vi "Insert Start Message.vi"(8 "error in (no error)":errorcluster, 10 "Start Time":timestamp, 11 "BehaviorData in":refnum<class "BehaviorData.lvclass">) -> (0 "error out":errorcluster, 3 "BehaviorData out":refnum<class "BehaviorData.lvclass">)   [LabVIEW 2010, in "BehaviorData.lvclass"]
uses:
  BehaviorData.lvclass
  Database/BehPrimary.ctl
  AcquireTraces/AcquireTraces.lvclass
  Database/StimulationPrimary.ctl
  <vilib>/addons/database/NI_Database_API.lvlib
  AcquistionObject/AcquistionObject.lvclass
panel:
  out "BehPK":T1
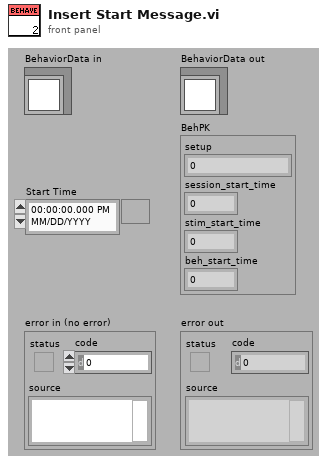
[diagram p1: front panel]
types:
  T1 = typedef "BehPrimary.ctl" = cluster{"setup":u8, "session_start_time":dbl, "stim_start_time":dbl, "beh_start_time":dbl}
  T2 = cluster{"setup":u8, "session_start_time":dbl, "stim_start_time":dbl, "beh_start_time":dbl, "beh_path":path, "beh_traces_type":string}
  T3 = typedef "NI_Database_API.lvlib/Conn ObjectReference.ctl" = refnum<k1>
  T4 = typedef "StimulationPrimary.ctl" = cluster{"setup":u8, "session_start_time":dbl, "stim_start_time":dbl}
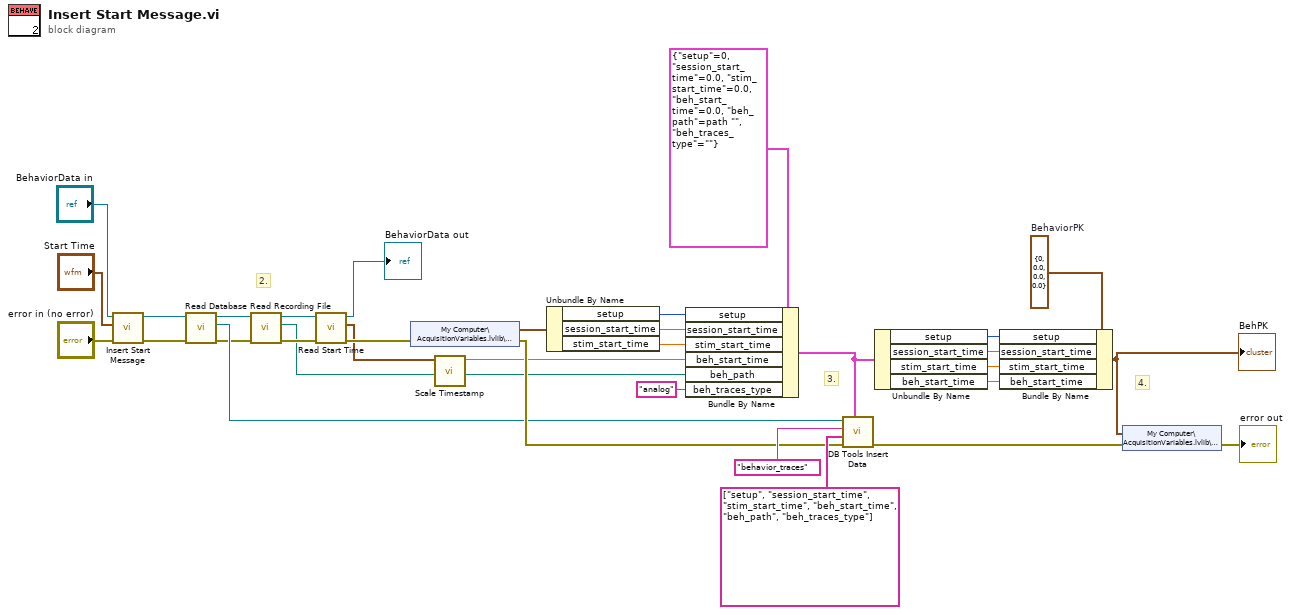
[diagram p0: block diagram]
diagram:
  w14 = T1 {"setup"=0, "session_start_time"=0.0, "stim_start_time"=0.0, "beh_start_time"=0.0}  # BehaviorPK
  # "4."
  # "2."
  # "3."
  n1 = call-parent "Insert Start Message.vi"("error in (no error)"="error in (no error)", "Start Time"="Start Time", "AcquireTraces in"="BehaviorData in") -> ("error out"=w10:errorcluster, "AcquireTraces out"=w11:refnum<class "BehaviorData.lvclass">)  [unwired: 7 in]
  n2 = call-dynamic "Read Database.vi"("error in (no error)"=w10, "AcquistionObject in"=w11) -> ("error out"=w13:errorcluster, "reference"=w17:T3, "AcquistionObject out"=w12:refnum<class "BehaviorData.lvclass">)  [unwired: 7 in]
  n3 = call-dynamic "Read Recording File.vi"("error in (no error)"=w13, "AcquistionObject in"=w12) -> ("error out"=w18:errorcluster, "Recording File"=w6:path, "AcquistionObject out"=w19:refnum<class "BehaviorData.lvclass">)  [unwired: 7 in]
  n4 = call-dynamic "Read Start Time.vi"("error in (no error)"=w18, "AcquistionObject in"=w19) -> ("error out"=w9:errorcluster, "Start Time"=w3:timestamp, "AcquistionObject out"=→"BehaviorData out":refnum<class "BehaviorData.lvclass">)  [unwired: 7 in]
  n5 = shared-variable "My Computer\\AcquisitionVariables.lvlib\\StimulationPK"(error in=w9) -> (w4:T4, error out=w22:errorcluster)
  n6 = call "Scale Timestamp.vi"("Time Stamp"=w3) -> ("Scaled timestamp"=w2:dbl)  [unwired: 10 in]
  n7 = Unbundle By Name(w4) -> ("setup"=w28:u8, "session_start_time"=w27:dbl, "stim_start_time"=w7:dbl)
  n8 = Bundle By Name(cluster=T2 {"setup"=0, "session_start_time"=0.0, "stim_start_time"=0.0, "beh_start_time"=0.0, "beh_path"=path "", "beh_traces_type"=""} ("Cluster"), "setup"=w28, "session_start_time"=w27, "stim_start_time"=w7, "beh_start_time"=w2, "beh_path"=w6, "beh_traces_type"="analog") -> (w26:T2)
  n9 = call <vilib>:"DB Tools Insert Data.vi"("data"=w26, "error in (no error)"=w22, "columns"=string[] ["setup", "session_start_time", "stim_start_time", "beh_start_time", "beh_path", "beh_traces_type"], "table"="behavior_traces", "connection reference"=w17) -> ("error out"=w20:errorcluster)  [unwired: 5 in, 1 out]
  n10 = Unbundle By Name(w26) -> ("setup"=w25:u8, "session_start_time"=w24:dbl, "stim_start_time"=w23:dbl, "beh_start_time"=w1:dbl)
  n11 = Bundle By Name(cluster=w14, "setup"=w25, "session_start_time"=w24, "stim_start_time"=w23, "beh_start_time"=w1) -> (w21:T1)
  "BehPK" <- w21
  n12 = shared-variable "My Computer\\AcquisitionVariables.lvlib\\BehaviorPK"(w21, error in=w20) -> (error out=→"error out":errorcluster)
